vi "Run All Tests.vi"() -> (0 "error out":errorcluster)   [LabVIEW 2013]
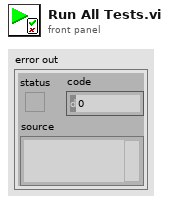
[diagram p1: front panel]
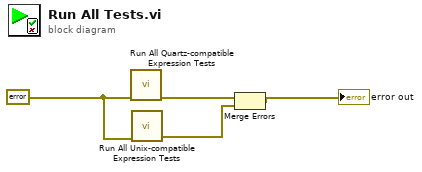
[diagram p0: block diagram]
diagram:
  w4 = errorcluster {"status"=FALSE, "code"=0, "source"=""} ("error in")
  n1 = call "Run All Quartz-compatible Expression Tests.vi"("error in"=w4) -> ("error out"=w3:errorcluster)  [unwired: 10 in]
  n2 = call "Run All Unix-compatible Expression Tests.vi"("error in"=w4) -> ("error out"=w1:errorcluster)  [unwired: 10 in]
  n3 = Merge Errors(w3, w1) -> (→"error out":errorcluster)
